vi "Volt Reader1.vi"() -> ()   [LabVIEW 2014]
uses:
  <vilib>/Utility/error.llb/DialogType.ctl
  <vilib>/_DAQmxBase/Internals/DAQmxBase Create Channel (AI-Voltage-Basic).vi
  <vilib>/_DAQmxBase/Internals/DAQmxBase Timing (Sample Clock).vi
  <vilib>/_DAQmxBase/Internals/DAQmxBase Read (Analog 2D DBL NChan NSamp).vi
panel:
  in  "units":i32(ring)=10348 items=["Volts"=10348, "From Custom Scale"=10065]
  in  "stop":bool
  out "Waveform Chart":dbl[][](graph)
  in  "physical channels":tag
  in  "maximum value":dbl=5.0 format="%0.2f"
  in  "minimum value":dbl=-5.0 format="%0.2f"
  in  "rate":i32=1000 caption="Sample Rate"
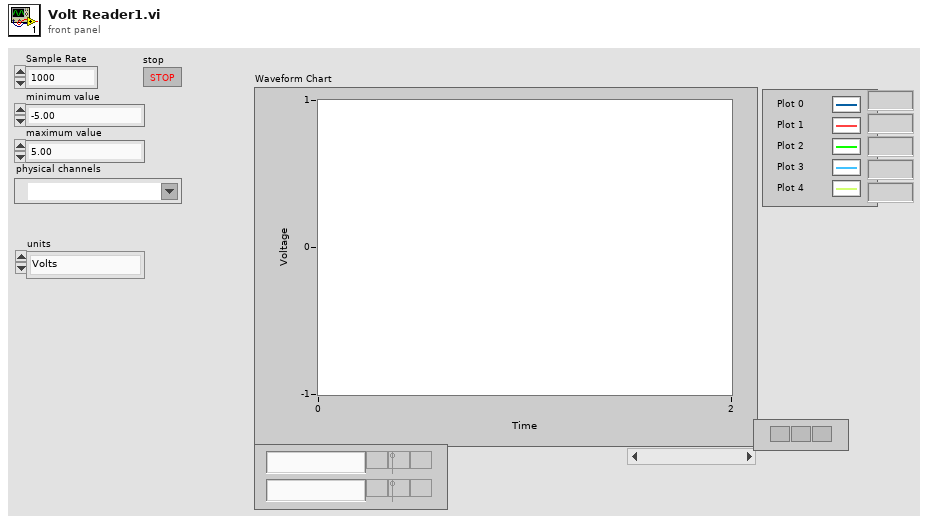
[diagram p1: front panel]
types:
  T1 = typedef "DialogType.ctl" = u16
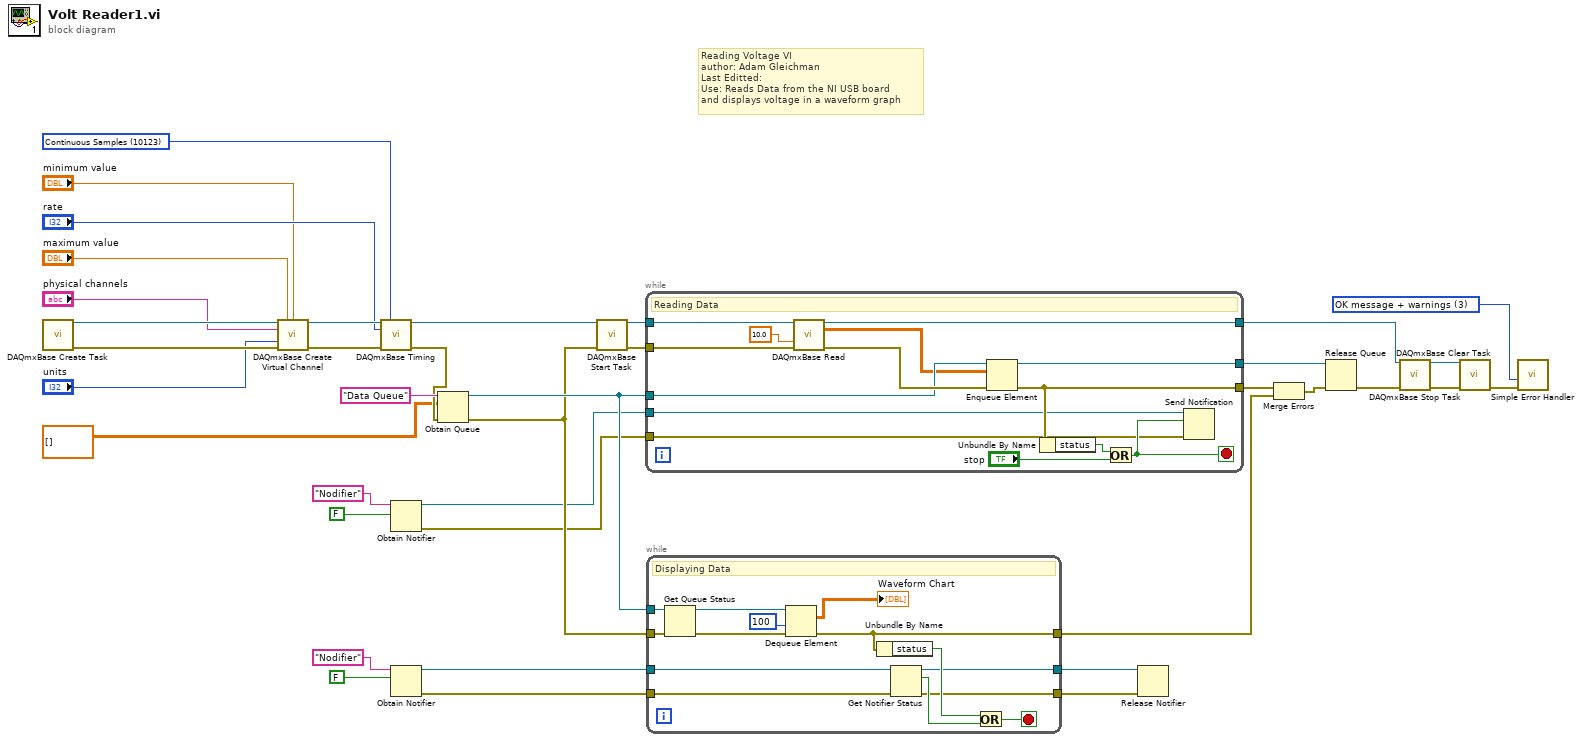
[diagram p0: block diagram]
diagram:
  w13 = 10123 items=["Finite Samples"=10178, "Continuous Samples"=10123, "Hardware Timed Single Point"=12522] ("sample mode")
  w15 = T1 3 items=["no dialog", "OK message", "continue or stop message", "OK message + warnings", "continue/stop + warnings"] ("type of dialog (OK msg:1)")
  # "Reading Voltage VI\nauthor: Adam Gleichman\nLast Editted: \nUse: Reads Data from the NI USB board\nand displays voltage in a waveform graph"
  n1 = call <vilib>:"DAQmxBase Create Task.vi"() -> ("task out"=w37:refnum<k21>, "error out"=w36:errorcluster)  [unwired: 5 in, 9 out]
  n2 = call-poly <vilib>:"DAQmxBase Create Virtual Channel.vi"("task in"=w37, "maximum value"="maximum value", "minimum value"="minimum value", "physical channels"="physical channels", "units"="units", "error in"=w36) -> ("task out"=w34:refnum<k21>, "error out"=w35:errorcluster)  [unwired: 3 in, 5 out]
  n3 = call-poly <vilib>:"DAQmxBase Timing.vi"("task/channels in"=w34, "sample mode"=w13, "rate"="rate", "error in"=w35) -> ("task out"=w1:refnum<k21>, "error out"=w33:errorcluster)  [unwired: 3 in, 7 out]
  n4 = Obtain Notifier(name (unnamed)="Nodifier", notification data type=FALSE) -> (notifier out=w9:refnum<notifier>, error out=w8:errorcluster)  [unwired: 2 in, 1 out]
  n5 = Obtain Notifier(name (unnamed)="Nodifier", notification data type=FALSE) -> (notifier out=w6:refnum<notifier>, error out=w4:errorcluster)  [unwired: 2 in, 1 out]
  n6 = Obtain Queue(name (unnamed)="Data Queue", element data type=dbl[][] [] ("data"), error in (no error)=w33) -> (queue out=w22:refnum<queue>, error out=w21:errorcluster)  [unwired: 2 in, 1 out]
  n7 = call <vilib>:"DAQmxBase Start Task.vi"("task/channels in"=w1, "error in"=w21) -> ("task out"=w31:refnum<k21>, "error out"=w32:errorcluster)  [unwired: 12 out]
  n8 = while "Data Reading Loop" {
    tunnel: w32 -> [w51]
    tunnel: w31 -> [w52]
    tunnel: w22 -> [w49]
    tunnel: [w46] -> w25
    tunnel: [w44] -> w24
    tunnel: [w42] -> w12
    tunnel: w9 -> [w40]
    tunnel: w8 -> [w39]
    stop <- w41 stop-if-true
    # "Reading Data"
    n9 = call-poly <vilib>:"DAQmxBase Read.vi"("task/channels in"=w52, "timeout"=10.0, "error in"=w51) -> ("task out"=w42:refnum<k21>, "data"=w47:dbl[][], "error out"=w50:errorcluster)  [unwired: 10 in]
    n10 = Enqueue Element(queue=w49, element=w47, error in (no error)=w50) -> (queue out=w46:refnum<queue>, error out=w44:errorcluster)  [unwired: 1 in, 1 out]
    n11 = Unbundle By Name(w44) -> ("status"=w43:bool)
    n12 = Or(x=w43, y="stop") -> (x .or. y?=w41:bool)
    n13 = Send Notification(notification=w41, notifier=w40, error in (no error)=w39) -> ()  [unwired: 2 out]
  }
  n14 = while {
    tunnel: w22 -> [w66]
    tunnel: w21 -> [w54]
    tunnel: [w64] -> w20
    tunnel: w6 -> [w61]
    tunnel: w4 -> [w60]
    tunnel: [w58] -> w2
    tunnel: [w57] -> w3
    stop <- w62 stop-if-true
    # "Displaying Data"
    n15 = Get Queue Status(queue=w66, error in (no error)=w54) -> (queue out=w55:refnum<queue>, error out=w53:errorcluster)  [unwired: 1 in, 6 out]
    n16 = Dequeue Element(queue=w55, timeout in ms (-1)=100, error in (no error)=w53) -> (element=→"Waveform Chart":dbl[][], error out=w64:errorcluster)  [unwired: 2 out]
    n17 = Unbundle By Name(w64) -> ("status"=w63:bool)
    n18 = Get Notifier Status(notifier=w61, error in (no error)=w60) -> (notifier out=w58:refnum<notifier>, current notification=w59:bool, error out=w57:errorcluster)  [unwired: 2 out]
    n19 = Or(x=w63, y=w59) -> (x .or. y?=w62:bool)
  }
  n20 = Release Notifier(notifier=w2, error in (no error)=w3) -> ()  [unwired: 1 in, 3 out]
  n21 = Merge Errors(w24, w20) -> (w23:errorcluster)
  n22 = Release Queue(queue=w25, error in (no error)=w23) -> (error out=w19:errorcluster)  [unwired: 1 in, 2 out]
  n23 = call <vilib>:"DAQmxBase Stop Task.vi"("task/channels in"=w12, "error in"=w19) -> ("task out"=w18:refnum<k21>, "error out"=w17:errorcluster)  [unwired: 12 in]
  n24 = call <vilib>:"DAQmxBase Clear Task.vi"("task in"=w18, "error in"=w17) -> ("error out"=w16:errorcluster)  [unwired: 13 in]
  n25 = call <vilib>:"Simple Error Handler.vi"("type of dialog (OK msg:1)"=w15, "error in (no error)"=w16) -> ()  [unwired: 3 in, 5 out]
